vi "Parse Data To Send.vi"(8 "Chosen Image Path":path, 9 "Chosen Text":string, 10 "Chosen Transmission Method":u16(ring)=3 items=["Barcode", "Wire", "Motor", "Touch", "Light", "Solenoid"], 11 "Chosen Data Type":u16(ring) items=["Text File", "Image File", "Image", "Text"]) -> ()   [LabVIEW 2026]
uses:
  Globals/QRCode VISA Global.vi
  Globals/Wire VISA Global.vi
  Globals/Motor VISA Global.vi
  Globals/Touch VISA Global.vi
  Globals/Light VISA Global.vi
  Globals/Solenoid VISA Global.vi
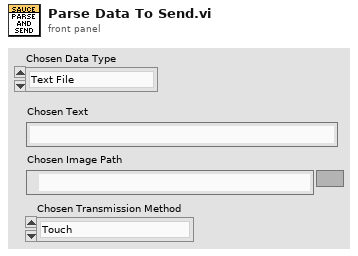
[diagram p1: front panel]
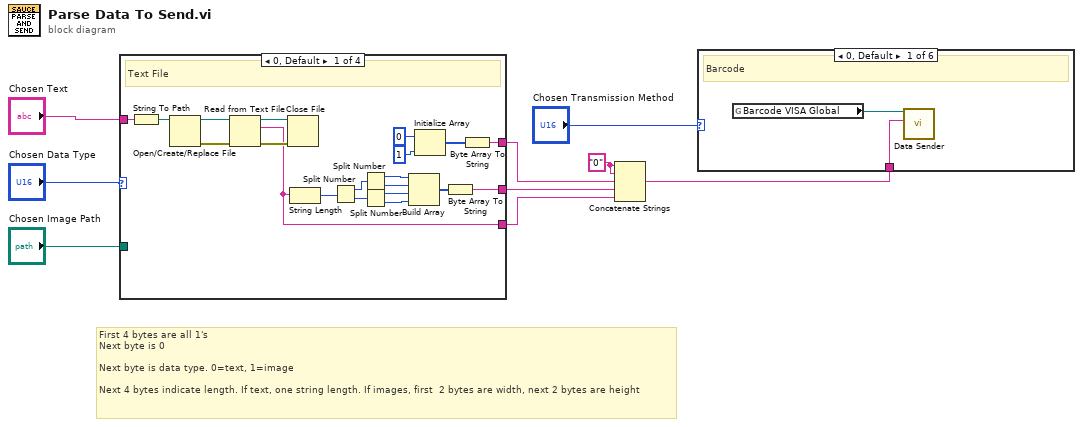
[diagram p0: block diagram]
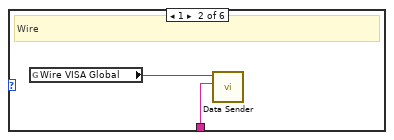
[diagram p2: hidden frame]
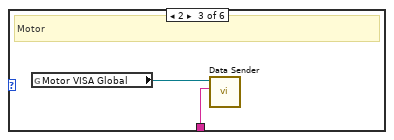
[diagram p3: hidden frame]
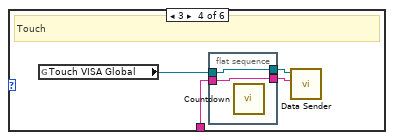
[diagram p4: hidden frame]
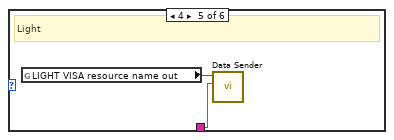
[diagram p5: hidden frame]
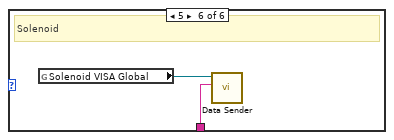
[diagram p6: hidden frame]
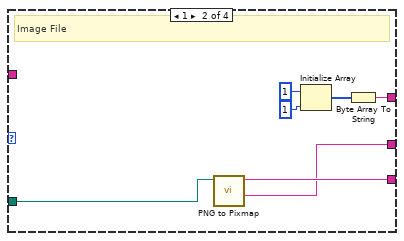
[diagram p7: hidden frame]
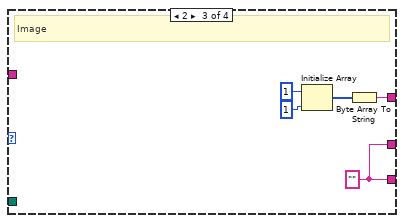
[diagram p8: hidden frame]
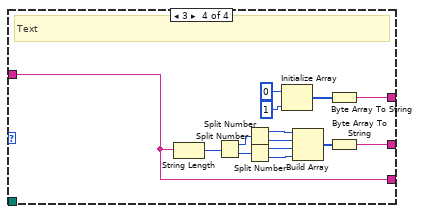
[diagram p9: hidden frame]
diagram:
  w1 = "0" ("string")
  # "First 4 bytes are all 1's\nNext byte is 0\n\nNext byte is data type. 0=text, 1=image\n\nNext 4 bytes indicate length. If text, one string length. If images, first  2 bytes are width, next 2 bytes are height"
  n1 = case shown="0, Default" "Chosen Data Type" {
    tunnel: "Chosen Text" -> [w29 _ _ w42]
    tunnel: [w23 w35 w41 w42] -> w5
    tunnel: "Chosen Image Path" -> [_ w36 _ _]
    tunnel: [w18 w30 w37 w53] -> w4
    tunnel: [w22 w34 w41 w43] -> w3
    frame 0, Default {
      # "Text File"
      n2 = String To Path(string=w29) -> (path=w28:path)
      n3 = Open/Create/Replace File(file path (use dialog)=w28) -> (refnum out=w26:refnum<file>, error out=w27:errorcluster)  [unwired: 5 in, 1 out]
      n4 = Read from Text File(file (use dialog)=w26, error in=w27) -> (refnum out=w24:refnum<file>, text=w23:string, error out=w25:errorcluster)  [unwired: 2 in, 1 out]
      n5 = Close File(refnum=w24, error in=w25) -> ()  [unwired: 2 out]
      n6 = String Length(string=w23) -> (length=w10:i32)
      n7 = Split Number(x=w10) -> (hi(x)=w12:u16, lo(x)=w13:u16)
      n8 = Split Number(x=w12) -> (hi(x)=w17:u8, lo(x)=w16:u8)
      n9 = Split Number(x=w13) -> (hi(x)=w14:u8, lo(x)=w15:u8)
      n10 = Build Array(w17, w16, w14, w15) -> (w11:u8[])
      n11 = Initialize Array(0 ("element"), 1 ("dimension size")) -> (w20:i32[])
      n12 = Byte Array To String(unsigned byte array=w11) -> (string=w22:string)
      n13 = Byte Array To String(unsigned byte array=w20) -> (string=w18:string)
    }
    frame 1 {
      # "Image File"
      n14 = call "PNG to Pixmap.vi"("path to PNG file"=w36) -> ("Size"=w34:string, "String"=w35:string)  [unwired: 9 in]
      n15 = Initialize Array(1 ("element"), 1 ("dimension size")) -> (w32:i32[])
      n16 = Byte Array To String(unsigned byte array=w32) -> (string=w30:string)
    }
    frame 2 {
      w41 = "" ("Chosen Text")
      # "Image"
      n17 = Initialize Array(1 ("element"), 1 ("dimension size")) -> (w39:i32[])
      n18 = Byte Array To String(unsigned byte array=w39) -> (string=w37:string)
    }
    frame 3 {
      # "Text"
      n19 = String Length(string=w42) -> (length=w51:i32)
      n20 = Split Number(x=w51) -> (hi(x)=w49:u16, lo(x)=w48:u16)
      n21 = Split Number(x=w49) -> (hi(x)=w44:u8, lo(x)=w45:u8)
      n22 = Split Number(x=w48) -> (hi(x)=w47:u8, lo(x)=w46:u8)
      n23 = Initialize Array(0 ("element"), 1 ("dimension size")) -> (w54:i32[])
      n24 = Build Array(w44, w45, w47, w46) -> (w50:u8[])
      n25 = Byte Array To String(unsigned byte array=w54) -> (string=w53:string)
      n26 = Byte Array To String(unsigned byte array=w50) -> (string=w43:string)
    }
  }
  n27 = Concatenate Strings(w1, w1, w4, w3, w5) -> (w2:string)
  n28 = case shown="0, Default" "Chosen Transmission Method" {
    tunnel: w2 -> [w57 w59 w60 w64 w68 w70]
    frame 0, Default {
      # "Barcode"
      n29 = global read "QRCode VISA Global.vi" "Barcode VISA Global"() -> (w56:refnum<visa-resource-name>)
      n30 = call "Data Sender.vi"("String To Send"=w57, "VISA resource name"=w56) -> ()  [unwired: 8 in, 2 out]
    }
    frame 1 {
      # "Wire"
      n31 = global read "Wire VISA Global.vi" "Wire VISA Global"() -> (w58:refnum<visa-resource-name>)
      n32 = call "Data Sender.vi"("String To Send"=w59, "VISA resource name"=w58) -> ()  [unwired: 8 in, 2 out]
    }
    frame 2 {
      # "Motor"
      n33 = global read "Motor VISA Global.vi" "Motor VISA Global"() -> (w61:refnum<visa-resource-name>)
      n34 = call "Data Sender.vi"("String To Send"=w60, "VISA resource name"=w61) -> ()  [unwired: 8 in, 2 out]
    }
    frame 3 {
      # "Touch"
      n35 = global read "Touch VISA Global.vi" "Touch VISA Global"() -> (w63:refnum<visa-resource-name>)
      n36 = flat-sequence {
        tunnel: [w67] -> w65
        tunnel: w64 -> [w67]
        tunnel: w63 -> [w66]
        tunnel: [w66] -> w62
        frame #0 {
          n37 = call "Countdown.vi"() -> ()  [unwired: 11 in, 1 out]
        }
      }
      n38 = call "Data Sender.vi"("String To Send"=w65, "VISA resource name"=w62) -> ()  [unwired: 8 in, 2 out]
    }
    frame 4 {
      # "Light"
      n39 = global read "Light VISA Global.vi" "LIGHT VISA resource name out"() -> (w69:refnum<visa-resource-name>)
      n40 = call "Data Sender.vi"("String To Send"=w68, "VISA resource name"=w69) -> ()  [unwired: 8 in, 2 out]
    }
    frame 5 {
      # "Solenoid"
      n41 = global read "Solenoid VISA Global.vi" "Solenoid VISA Global"() -> (w71:refnum<visa-resource-name>)
      n42 = call "Data Sender.vi"("String To Send"=w70, "VISA resource name"=w71) -> ()  [unwired: 8 in, 2 out]
    }
  }
